vi "ryTimerEx Queue One Shot.vi"() -> ()   [LabVIEW 2020]
uses:
  3122cb75-6530-49f8-9864-937ee694b227.vi
panel:
  out "Element out":string
  out "Time Ellapsed (ms)":u32
  out "Error":errorcluster
  # "Waits 5 seconds\nbefore receiving\nand \"EXIT\" element\nto stop this VI."
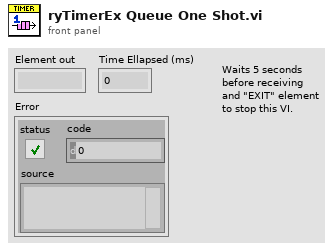
[diagram p1: front panel]
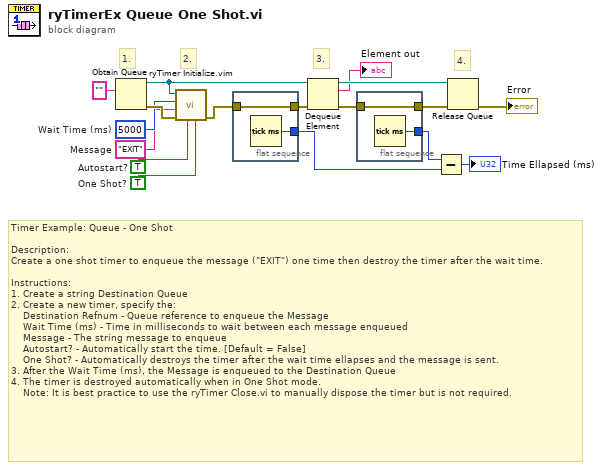
[diagram p0: block diagram]
diagram:
  w10 = TRUE  # One Shot?
  w13 = TRUE  # Autostart?
  w14 = "EXIT"  # Message
  w15 = u32 5000  # Wait Time (ms)
  # "Timer Example: Queue - One Shot\n\nDescription:\nCreate a one shot timer to enqueue the message (\"EXIT\") one time then destroy the timer after the wait time.\n\nInstructions:\n1. Create a string Destination Queue\n2. Create a new timer, specify the:\n    Destination Refnum - Queue reference to enqueue the Message\n    Wait Time (ms) - Time in milliseconds to wait between each message enqueued\n    Message - The string message to enqueue\n    Autostart? - Automatically start the time. [Default = False]\n    One Shot? - Automatically destroys the timer after the wait time ellapses and the message is sent.\n3. After the Wait Time (ms), the Message is enqueued to the Destination Queue\n4. The timer is destroyed automatically when in One Shot mode.\n    Note: It is best practice to use the ryTimer Close.vi to manually dispose the timer but is not required."
  # "3."
  # "4."
  # "2."
  # "1."
  n1 = Obtain Queue(element data type="") -> (queue out=w12:refnum<queue>, error out=w16:errorcluster)  [unwired: 4 in, 1 out]
  n2 = call "ryTimer Initialize.vim"("One Shot? (F=Repeat)"=w10, "Autostart? (F)"=w13, "error in (no error)"=w16, "Message"=w14, "Wait Time (ms)"=w15, "Destination Refnum [Q,UE,Any]"=w12) -> ("error out"=w9:errorcluster)  [unwired: 4 in, 1 out]
  n3 = flat-sequence {
    tunnel: w9 -> [w19]
    tunnel: [w19] -> w8
    tunnel: [w18] -> w5
    frame #0 {
      n4 = Tick Count (ms)() -> (millisecond timer value=w18:u32)
    }
  }
  n5 = Dequeue Element(queue=w12, error in (no error)=w8) -> (queue out=w3:refnum<queue>, element=→"Element out":string, error out=w7:errorcluster)  [unwired: 1 in, 1 out]
  n6 = flat-sequence {
    tunnel: w7 -> [w21]
    tunnel: [w21] -> w1
    tunnel: [w20] -> w6
    frame #0 {
      n7 = Tick Count (ms)() -> (millisecond timer value=w20:u32)
    }
  }
  n8 = Subtract(x=w6, y=w5) -> (x-y=→"Time Ellapsed (ms)":u32)
  n9 = Release Queue(queue=w3, error in (no error)=w1) -> (error out=→"Error":errorcluster)  [unwired: 1 in, 2 out]
